vi "create_morph_kernel.vi"(11 "kernel size":dbl) -> (3 "kernel":dbl[][](array[numeric]))   [LabVIEW 2017]
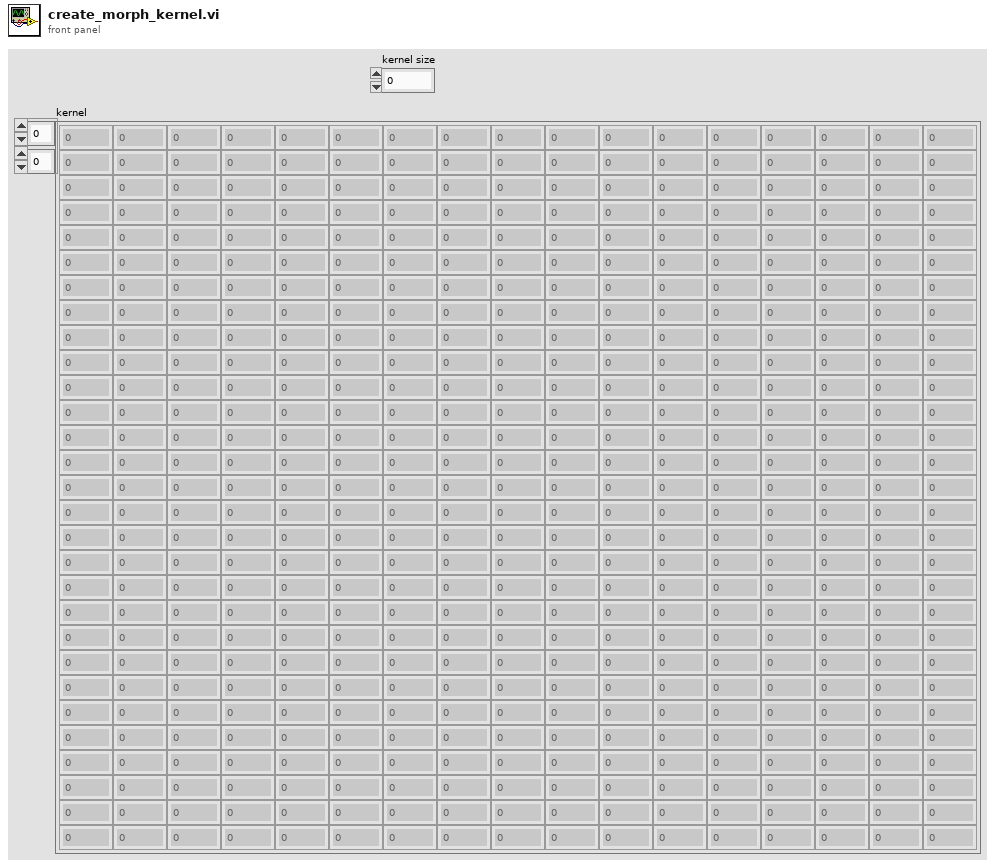
[diagram p1: front panel]
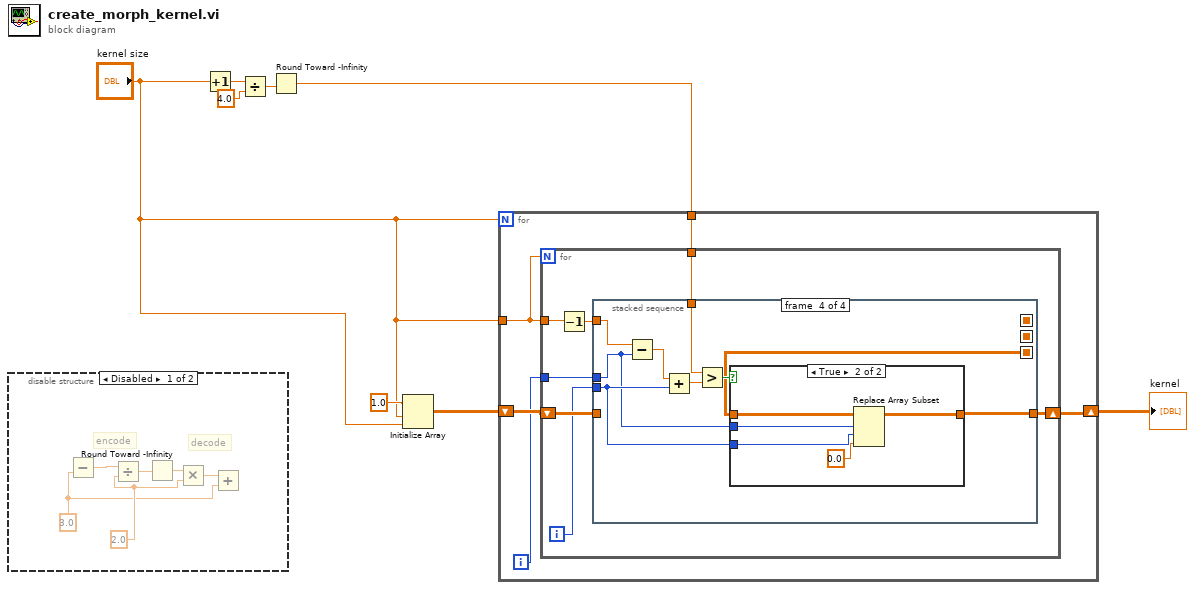
[diagram p0: block diagram]
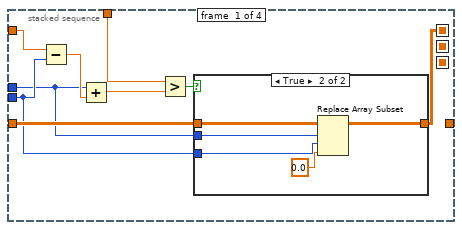
[diagram p3: hidden frame]
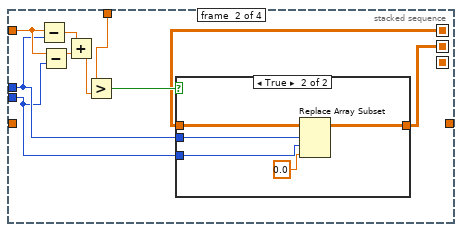
[diagram p5: hidden frame]
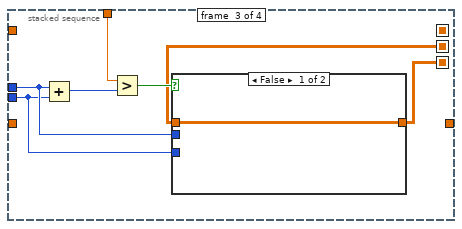
[diagram p7: hidden frame]
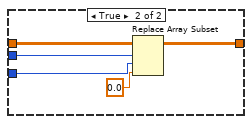
[diagram p8: hidden frame]
diagram:
  n1 = disable-structure shown="Disabled" {
    frame Disabled {
      w12 = 2.0 ("y")
      w10 = 3.0 ("y")
      # "decode"
      # "encode"
      n2 = Subtract(y=w10) -> (x=w9:dbl, x-y=w15:dbl)
      n3 = Divide(x=w15, y=w12) -> (x/y=w14:dbl)
      n4 = Round Toward -Infinity(1:w14) -> (0:w13:dbl)
      n5 = Multiply(x=w13, y=w12) -> (x*y=w11:dbl)
      n6 = Add(x=w11, y=w10) -> ()  [unwired: 1 out]
    }
    frame Enabled {
    }
  }
  n7 = Increment(x="kernel size") -> (x+1=w6:dbl)
  n8 = Divide(x=w6, y=4.0) -> (x/y=w8:dbl)
  n9 = Round Toward -Infinity(1:w8) -> (0:w2:dbl)
  n10 = Initialize Array(1.0 ("element"), "kernel size", "kernel size") -> (w3:dbl[][])
  n11 = for {
    N: "kernel size" -> [_]
    shift-right: [w19] -> w4
    shift-left: w3 -> [w20]
    tunnel: w2 -> [w17]
    tunnel: "kernel size" -> [w16]
    i -> [w18]
    n12 = for {
      N: w16 -> [_]
      shift-right: [w26] -> w19
      shift-left: w20 -> [w27]
      tunnel: w18 -> [w24]
      tunnel: w17 -> [w23]
      tunnel: w16 -> [w22]
      i -> [w25]
      n13 = Decrement(x=w22) -> (x-1=w21:dbl)
      n14 = stacked-sequence {
        seq-local: [w32 _ _ _] -> [_ w49 _ _]
        seq-local: [_ w48 _ _] -> [_ _ w62 _]
        seq-local: [_ _ w61 _] -> [_ _ _ w75]
        tunnel: w27 -> [w35 _ _ _]
        tunnel: [_ _ _ w78] -> w26
        tunnel: w25 -> [w30 w45 w59 w77]
        tunnel: w24 -> [w28 w46 w60 w72]
        tunnel: w23 -> [w33 w50 w63 w76]
        tunnel: w21 -> [w31 w47 _ w74]
        frame #0 {
          n15 = Subtract(x=w31, y=w30) -> (x-y=w29:dbl)
          n16 = Add(x=w28, y=w29) -> (x+y=w36:dbl)
          n17 = Greater?(x=w33, y=w36) -> (0:w34:bool)
          n18 = case shown="True" w34 {
            tunnel: w35 -> [w37 w42]
            tunnel: [w37 w41] -> w32
            tunnel: w30 -> [_ w39]
            tunnel: w28 -> [_ w38]
            frame False {
            }
            frame True {
              n19 = Replace Array Subset(array=w42, new element=0.0 ("new element/subarray"), index (row)=w38, index (col)=w39) -> (w41:dbl[][])
            }
          }
        }
        frame #1 {
          n20 = Subtract(x=w47, y=w46) -> (x-y=w44:dbl)
          n21 = Subtract(x=w47, y=w45) -> (x-y=w43:dbl)
          n22 = Add(x=w44, y=w43) -> (x+y=w52:dbl)
          n23 = Greater?(x=w50, y=w52) -> (0:w51:bool)
          n24 = case shown="True" w51 {
            tunnel: w49 -> [w53 w58]
            tunnel: [w53 w57] -> w48
            tunnel: w45 -> [_ w55]
            tunnel: w46 -> [_ w54]
            frame False {
            }
            frame True {
              n25 = Replace Array Subset(array=w58, new element=0.0 ("new element/subarray"), index (row)=w54, index (col)=w55) -> (w57:dbl[][])
            }
          }
        }
        frame #2 {
          n26 = Add(x=w60, y=w59) -> (x+y=w65:i32)
          n27 = Greater?(x=w63, y=w65) -> (0:w64:bool)
          n28 = case shown="False" w64 {
            tunnel: w62 -> [w66 w71]
            tunnel: [w66 w70] -> w61
            tunnel: w59 -> [_ w68]
            tunnel: w60 -> [_ w67]
            frame False {
            }
            frame True {
              n29 = Replace Array Subset(array=w71, new element=0.0 ("new element/subarray"), index (row)=w67, index (col)=w68) -> (w70:dbl[][])
            }
          }
        }
        frame #3 {
          n30 = Subtract(x=w74, y=w72) -> (x-y=w73:dbl)
          n31 = Add(x=w73, y=w77) -> (x+y=w80:dbl)
          n32 = Greater?(x=w76, y=w80) -> (0:w79:bool)
          n33 = case shown="True" w79 {
            tunnel: w75 -> [w81 w86]
            tunnel: [w81 w85] -> w78
            tunnel: w77 -> [_ w83]
            tunnel: w72 -> [_ w82]
            frame False {
            }
            frame True {
              n34 = Replace Array Subset(array=w86, new element=0.0 ("new element/subarray"), index (row)=w82, index (col)=w83) -> (w85:dbl[][])
            }
          }
        }
      }
    }
  }
  "kernel" <- w4
